vi "Get Pattern.vi"(11 "File Interface in":refnum<class "File Interface.lvclass">) -> (2 "file extension":string)   [LabVIEW 2018, in "ImportExport.lvlib" / "File Interface.lvclass"]
uses:
  Switch Configuration.llb/File Interface.lvclass
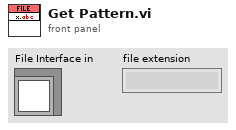
[diagram p1: front panel]
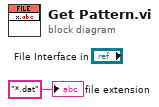
[diagram p0: block diagram]
diagram:
  "file extension" <- "*.dat" ("file extension")
